vi "Assign 3 Car Wiper (1).vi"() -> ()   [LabVIEW 2021]
panel:
  out "Car Wipers":bool
  in  "Wiper Switch":bool
  in  "Ignition Switch":bool
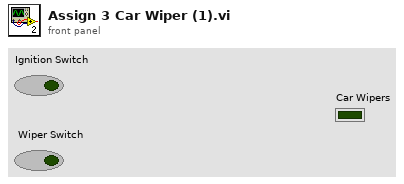
[diagram p1: front panel]
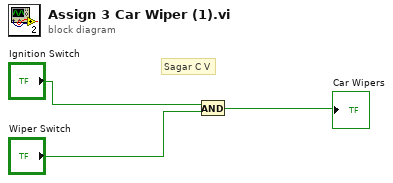
[diagram p0: block diagram]
diagram:
  # "Sagar C V"
  n1 = And(x="Ignition Switch", y="Wiper Switch") -> (x .and. y?=→"Car Wipers":bool)
